vi "Load Async.vi"(7 "Deck ID":string, 8 "error in (no error)":errorcluster, 9 "Message Queue":refnum<queue>, 10 "Path":path, 11 "Audio Data Reference":refnum<data-value>) -> (0 "error out":errorcluster)   [LabVIEW 2019, in "Audio File Input.lvlib"]
doc: "This VI loads an audio track, placing the audio data into the specified DVR.\n\n<b>Priority:</b> Background\n<b>Execution System:</b> Other 1"
uses:
  Audio File Input.lvlib
  Messaging/Message Cluster.ctl
  Track Info/Track Info FGV Enum.ctl
  <vilib>/Analysis/5stat.llb/RMS (DBL).vi
  Globals/Constants.vi
  Messaging/Messaging.lvlib
  <vilib>/Analysis/NI_AALPro.lvlib
  Audio Processing/Audio Processing.lvlib
  Globals/Globals.lvlib
  Track Info/Track Info.lvlib
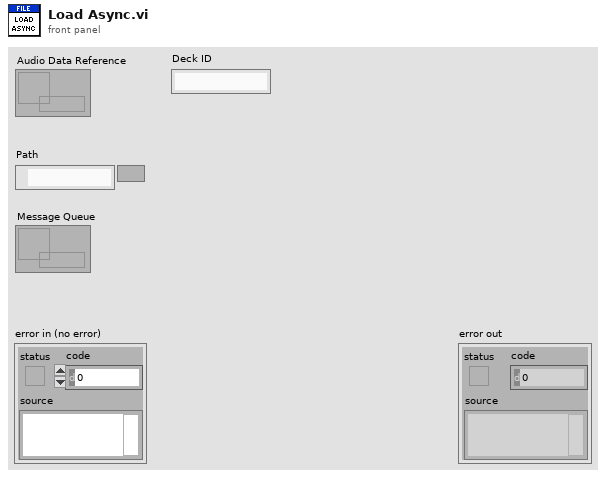
[diagram p1: front panel]
types:
  T1 = typedef "Track Info.lvlib/Track Info FGV Enum.ctl" = enum16{"Init", "Update Track", "Update Multiple Tracks", "Get Track", "Get Multiple Tracks"}
  T2 = typedef "Messaging.lvlib/Message Cluster.ctl" = cluster{"Event":string, "Source":string, "Target":string, "Data":variant}
  T3 = typedef "Track Info.lvlib/Track Info.ctl" = cluster{"Path":path, "Length (Samples)":i32, "Channels":i32, "Sample Rate (Hz)":i32, "BPM":dbl, "Cue Points (Samples)":i32[]}
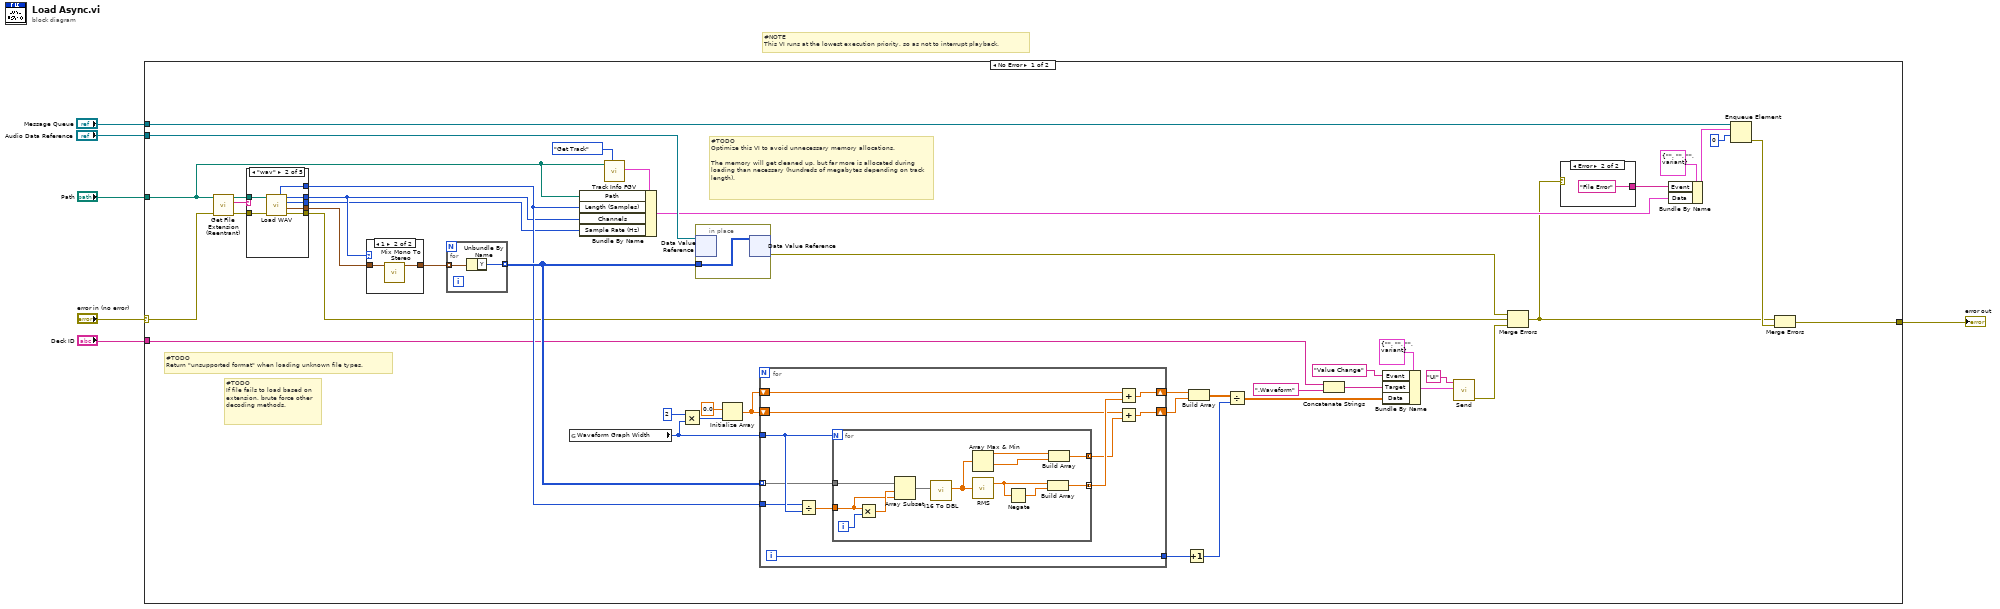
[diagram p0: block diagram]
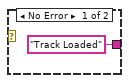
[diagram p3: hidden frame]
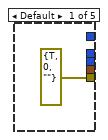
[diagram p4: hidden frame]
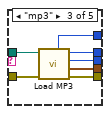
[diagram p5: hidden frame]
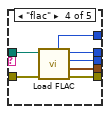
[diagram p6: hidden frame]
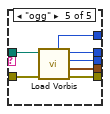
[diagram p7: hidden frame]
diagram:
  # "#NOTE\nThis VI runs at the lowest execution priority, so as not to interrupt playback."
  n1 = case shown="No Error" "error in (no error)" {
    selector: "error in (no error)" -> [w26 w111]
    tunnel: [w21 w111] -> w5
    tunnel: "Path" -> [w10 _]
    tunnel: "Message Queue" -> [w50 _]
    tunnel: "Audio Data Reference" -> [w46 _]
    tunnel: "Deck ID" -> [w12 _]
    frame No Error {
      # "#TODO\nOptimize this VI to avoid unnecessary memory allocations.\n\nThe memory will get cleaned up, but far more is allocated during loading than necessary (hundreds of megabytes depending on track length)."
      # "#TODO\nIf file fails to load based on extension, brute force other decoding methods."
      # "#TODO\nReturn \"unsupported format\" when loading unknown file types."
      n2 = call "Get File Extension (Reentrant).vi"("error in (no error)"=w26, "file"=w10) -> ("error out"=w25:errorcluster, "lowercase file extension"=w24:string, "dup file"=w23:path)  [unwired: 5 in, 2 out]
      n3 = case shown="\"wav\"" w24 {
        tunnel: w23 -> [_ w62 w70 w77 w84]
        tunnel: w25 -> [_ w63 w69 w76 w83]
        tunnel: [errorcluster {"status"=TRUE, "code"=0, "source"=""} ("error out") w58 w68 w75 w82] -> w11
        tunnel: [_ w59 w67 w74 w81] -> w14
        tunnel: [_ w61 w66 w73 w80] -> w9
        tunnel: [_ w60 w65 w72 w79] -> w8
        tunnel: [_ w57 w64 w71 w78] -> w13
        frame Default {
        }
        frame "wav" {
          n4 = call "Load WAV.vi"("error in (no error)"=w63, "Path"=w62) -> ("error out"=w58:errorcluster, "data"=w59:waveform(i16)[], "Sample Rate (Hz)"=w60:i32, "Channels"=w61:i32, "Length (Samples)"=w57:i32)  [unwired: 5 in]
        }
        frame "mp3" {
          n5 = call "Load MP3.vi"("error in (no error)"=w69, "Path"=w70) -> ("error out"=w68:errorcluster, "data"=w67:waveform(i16)[], "Sample Rate (Hz)"=w65:i32, "Channels"=w66:i32, "Length (Samples)"=w64:i32)  [unwired: 5 in]
        }
        frame "flac" {
          n6 = call "Load FLAC.vi"("error in (no error)"=w76, "Path"=w77) -> ("error out"=w75:errorcluster, "data"=w74:waveform(i16)[], "Sample Rate (Hz)"=w72:i32, "Channels"=w73:i32, "Length (Samples)"=w71:i32)  [unwired: 5 in]
        }
        frame "ogg" {
          n7 = call "Load Vorbis.vi"("error in (no error)"=w83, "Path"=w84) -> ("error out"=w82:errorcluster, "data"=w81:waveform(i16)[], "Sample Rate (Hz)"=w79:i32, "Channels"=w80:i32, "Length (Samples)"=w78:i32)  [unwired: 5 in]
        }
      }
      n8 = case shown="1" w9 {
        tunnel: w14 -> [w51 w53]
        tunnel: [w51 w52] -> w18
        frame Default {
        }
        frame 1 {
          n9 = call "Mix Mono To Stereo.vi"("Audio Data"=w53) -> ("Audio Data Out"=w52:waveform(i16)[])  [unwired: 10 in]
        }
      }
      n10 = for {
        tunnel: w18 -> [w110] mode=indexing
        tunnel: [w109] -> w27 mode=indexing
        n11 = Unbundle By Name(w110) -> ("Y"=w109:i16[])
      }
      n12 = global read "Constants.vi" "Waveform Graph Width"() -> (w15:i32)
      n13 = call "Track Info FGV.vi"("Track Info FGV Enum"=Track_Info_FGV_Enum."Get Track", "Track Path"=w10) -> ("Track Info Out"=w19:T3)  [unwired: 6 in, 3 out]
      n14 = Bundle By Name(cluster=w19, "Path"=w10, "Length (Samples)"=w13, "Channels"=w9, "Sample Rate (Hz)"=w8) -> (w28:T3)
      n15 = Multiply(x=2, y=w15) -> (x*y=w16:i32)
      n16 = in-place {
        in-place-border: w27 -> [w108]
        n17 = in-place-dvr #1(w46) -> ()  [unwired: 2 out]
        n18 = in-place-dvr #1(w108) -> (w45:errorcluster)  [unwired: 1 out]
      }
      n19 = Initialize Array(0.0 ("element"), w16) -> (w43:dbl[])
      n20 = for {
        tunnel: w27 -> [w86] mode=indexing
        tunnel: w15 -> [w95]
        shift-right: [w90] -> w42
        shift-left: w43 -> [w93]
        shift-right: [w89] -> w41
        shift-left: w43 -> [w92]
        tunnel: w13 -> [w87]
        tunnel: [w85] -> w39
        i -> [w85]
        n21 = Divide(x=w87, y=w95) -> (x/y=w88:dbl)
        n22 = for {
          N: w95 -> [_]
          tunnel: w86 -> [w107]
          tunnel: [w100] -> w91 mode=concatenating
          tunnel: [w99] -> w94 mode=concatenating
          tunnel: w88 -> [w98]
          i -> [w106]
          n23 = Multiply(x=w98, y=w106) -> (x*y=w105:dbl)
          n24 = Array Subset(array=w107, index=w105, length=w98) -> (w97:i16[])
          n25 = call "I16 To DBL.vi"("Audio Data (1D I16)"=w97) -> ("Audio Data (1D DBL)"=w96:dbl[])  [unwired: 9 in, 1 out]
          n26 = Array Max & Min(array=w96) -> (max value=w102:dbl, min value=w101:dbl)  [unwired: 2 out]
          n27 = call-poly <vilib>:"RMS.vi"("X"=w96) -> ("rms value"=w104:dbl)  [unwired: 1 out]
          n28 = Negate(x=w104) -> (-x=w103:dbl)
          n29 = Build Array(w104, w103) -> (w99:dbl[])
          n30 = Build Array(w102, w101) -> (w100:dbl[])
        }
        n31 = Add(x=w93, y=w94) -> (x+y=w90:dbl[])
        n32 = Add(x=w92, y=w91) -> (x+y=w89:dbl[])
      }
      n33 = Increment(x=w39) -> (x+1=w38:i32)
      n34 = Build Array(w42, w41) -> (w40:dbl[][])
      n35 = Divide(x=w40, y=w38) -> (x/y=w30:dbl[][])
      n36 = Concatenate Strings(w12, ".Waveform" ("string")) -> (w34:string)
      n37 = Bundle By Name(cluster=T2 {"Event"="", "Source"="", "Target"="", "Data"=variant} ("Message"), "Event"="Value Change", "Target"=w34, "Data"=w30) -> (w31:T2)
      n38 = call "Send.vi"("Message"=w31, "Queue Name"="UI") -> ("error out"=w29:errorcluster)  [unwired: 9 in]
      n39 = Merge Errors(w45, w11, w29) -> (w7:errorcluster)
      n40 = case shown="Error" w7 {
        tunnel: ["Track Loaded" ("Type") "File Error" ("Type")] -> w47
        frame No Error {
        }
        frame Error {
        }
      }
      n41 = Bundle By Name(cluster=T2 {"Event"="", "Source"="", "Target"="", "Data"=variant} ("element"), "Event"=w47, "Data"=w28) -> (w48:T2)
      n42 = Enqueue Element(queue=w50, element=w48, timeout in ms (-1)=0) -> (error out=w22:errorcluster)  [unwired: 1 in, 2 out]
      n43 = Merge Errors(w7, w22) -> (w21:errorcluster)
    }
    frame Error {
    }
  }
  "error out" <- w5
